vi "mod_acceleratetopoint.vi"(0 "Startpoint":dbl=2.0, 1 "Endpoint":dbl=1.0, 2 "tolerance":dbl=0.001, 3 "divisor":dbl=2.0, 4 "reset? (F)":bool) -> (5 "Next Point":dbl=1.0, 6 "move complete":bool=TRUE)   [LabVIEW 2020, in "niDMT.lvlib"]
uses:
  <vilib>/addons/Modulation/niDMT.lvlib
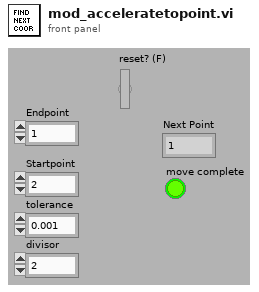
[diagram p1: front panel]
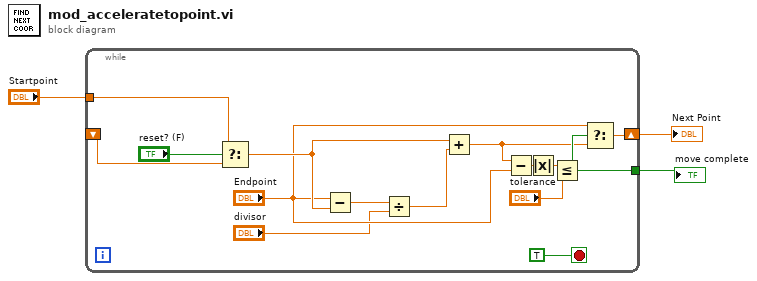
[diagram p0: block diagram]
diagram:
  n1 = while {
    shift-right: [w6] -> w3
    shift-left: _ -> [w16]
    tunnel: [w9] -> w2
    tunnel: "Startpoint" -> [w4]
    stop <- TRUE stop-if-true
    n2 = Select(t=w4, s="reset? (F)", f=w16) -> (s? t:f=w13:dbl)
    n3 = Subtract(x="Endpoint", y=w13) -> (x-y=w15:dbl)
    n4 = Divide(x=w15, y="divisor") -> (x/y=w14:dbl)
    n5 = Add(x=w13, y=w14) -> (x+y=w7:dbl)
    n6 = Subtract(x=w7, y="Endpoint") -> (x-y=w12:dbl)
    n7 = Absolute Value(x=w12) -> (abs(x)=w11:dbl)
    n8 = Less Or Equal?(x=w11, y="tolerance") -> (x <= y?=w9:bool)
    n9 = Select(t="Endpoint", s=w9, f=w7) -> (s? t:f=w6:dbl)
  }
  "Next Point" <- w3
  "move complete" <- w2
